vi "LVDimInterface.dim_unfold_data_info.vi"(0 "rawData":i8[](array[numeric]), 5 "error in (no error)":errorcluster) -> (8 "quality":i32, 10 "timeStamp":dbl, 11 "refNumType":i32, 12 "callBackID":i32, 13 "serviceID":u32, 14 "data":i8[](array[numeric]), 15 "serviceName":string, 16 "typeDescriptor":string, 17 "no link":bool, 18 "callBackType":i32, 19 "error out":errorcluster)   [LabVIEW 2014, in "LVDimInterface.lvlib"]
doc: "Unfolds the raw data from the DIMWrapper dll and gets information about a DIM (command) service. For optimum performance, please use the VI ...dim_unfold_data.vi.\n\nHistory: 13-FEB-2006, Dietrich Beck\n\nCopyright (C)\nGesellschaft für Schwerionenforschung, GSI\nPlanckstr. 1\n64291 Darmstadt\nGermany\n\nContact: D.Beck@gsi.de \n\nThis program is free software; you can redistribute it and/or modify it under the terms of the \nGNU General Public License as published by the Free Software Foundation; either version 2 of the license, or (at your option) any later version.\n\nThis program is distributed in the hope that it will be useful, but WITHOUT ANY WARRANTY; without even the implied warranty of MERCHANTABILITY or FITNESS FOR A PARTICULAR PURPOSE. See the GNU General License for more details (http://www.gnu.org).\n\nGesellschaft für Schwerionenforschung, GSI\nPlanckstr. 1, 64291 Darmstadt, Germany\nFor all questions and ideas contact D. Beck.\nLast update: 16-DEC-2005"
uses:
  LVDimInterface.lvlib
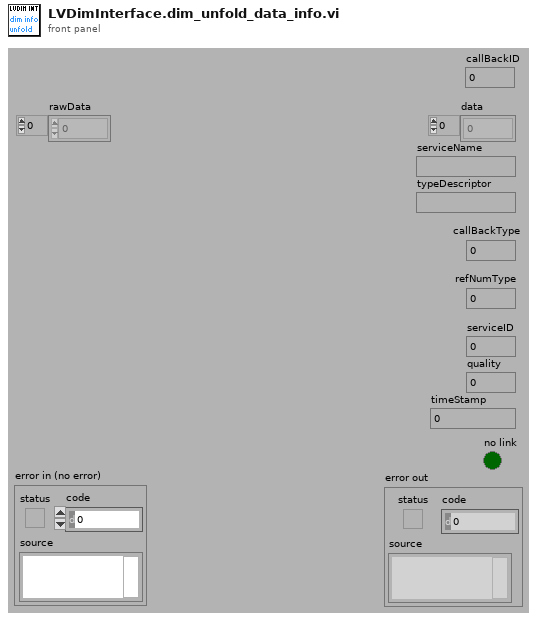
[diagram p1: front panel]
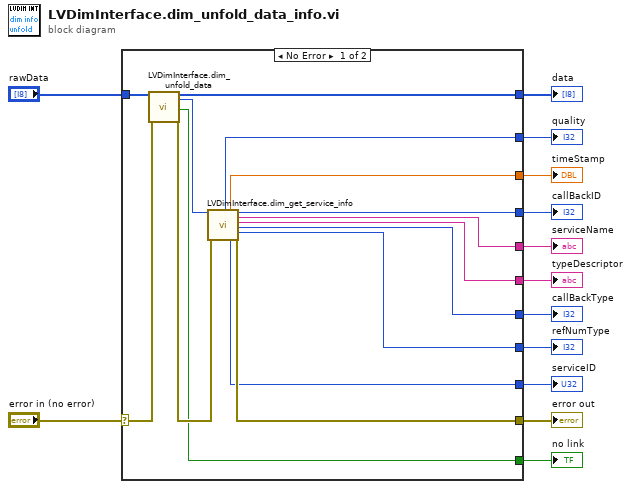
[diagram p0: block diagram]
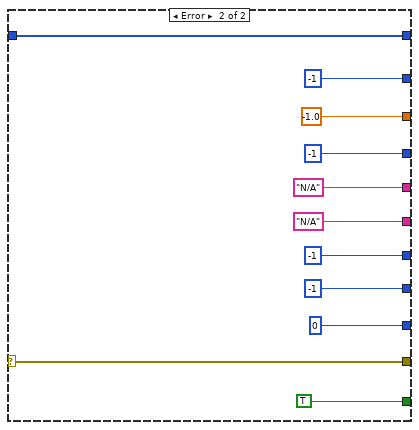
[diagram p2: hidden frame]
diagram:
  n1 = case shown="No Error" "error in (no error)" {
    selector: "error in (no error)" -> [w20 w35]
    tunnel: [w24 -1 ("refNumType")] -> w13
    tunnel: [w23 u32 0 ("serviceID")] -> w12
    tunnel: [w25 -1 ("callBackType")] -> w11
    tunnel: [w26 "N/A" ("typeDescriptor")] -> w10
    tunnel: [w28 w35] -> w9
    tunnel: [w27 "N/A" ("serviceName")] -> w7
    tunnel: "rawData" -> [w21 w33]
    tunnel: [w16 w33] -> w5
    tunnel: [w22 -1 ("callBackID (out)")] -> w4
    tunnel: [w17 TRUE ("no link")] -> w3
    tunnel: [w15 -1 ("quality")] -> w2
    tunnel: [w14 -1.0 ("timeStamp")] -> w1
    frame No Error {
      n2 = call "LVDimInterface.dim_unfold_data.vi"("rawData"=w21, "error in (no error)"=w20) -> ("data"=w16:i8[], "callBackID"=w18:i32, "no link"=w17:bool, "error out"=w19:errorcluster)  [unwired: 14 in]
      n3 = call "LVDimInterface.dim_get_service_info.vi"("callBackID"=w18, "error in (no error)"=w19) -> ("quality"=w15:i32, "timeStamp"=w14:dbl, "serviceID"=w23:u32, "callBackID (out)"=w22:i32, "serviceName"=w27:string, "typeDescriptor"=w26:string, "callBackType"=w25:i32, "refNumType"=w24:i32, "error out"=w28:errorcluster)  [unwired: 8 in, 1 out]
    }
    frame Error {
    }
  }
  "error out" <- w9
  "data" <- w5
  "typeDescriptor" <- w10
  "refNumType" <- w13
  "serviceID" <- w12
  "callBackType" <- w11
  "serviceName" <- w7
  "callBackID" <- w4
  "no link" <- w3
  "quality" <- w2
  "timeStamp" <- w1
